vi "Channel Index to Channel Type.vi"(10 "Rx channel range":cluster{"minimum":i32, "maximum":i32}={"minimum"=0, "maximum"=15}, 11 "hardware channel":i32) -> (2 "custom device channel type":T1, 3 "GUID for hardware channel type":string)   [LabVIEW 2020, in "Communication Bus Template Scripting.lvlib"]
uses:
  Communication Bus Template Scripting.lvlib
  <vilib>/NI VeriStand/Custom Device API/Custom Device Channel Type.ctl
  Constants.vi
  <vilib>/NI VeriStand/Custom Device API/Custom Device API.lvlib
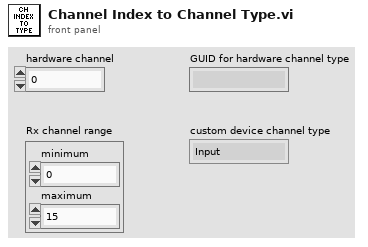
[diagram p1: front panel]
types:
  T1 = typedef "Custom Device API.lvlib/Custom Device Channel Type.ctl" = enum16{"Input", "Output"}
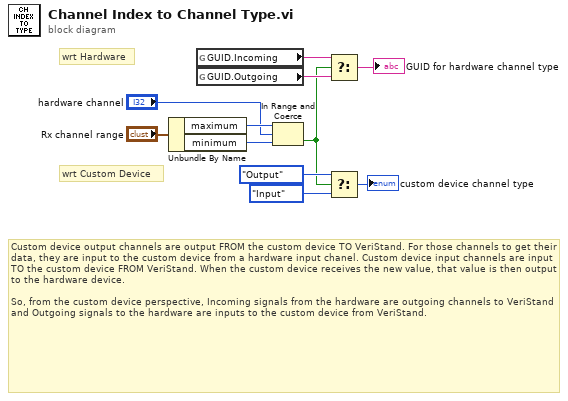
[diagram p0: block diagram]
diagram:
  # "wrt Custom Device"
  # "wrt Hardware"
  # "Custom device output channels are output FROM the custom device TO VeriStand. For those channels to get their data, they are input to the custom device from a hardware input chanel. Custom device input channels are input TO the custom device FROM VeriStand. When the custom device receives the new value, that value is then output to the hardware device.\n \nSo, from the custom device perspective, Incoming signals from the hardware are outgoing channels to VeriStand and Outgoing signals to the hardware are inputs to the custom device from VeriStand."
  n1 = Unbundle By Name("Rx channel range") -> ("maximum"=w7:i32, "minimum"=w6:i32)
  n2 = global read "Constants.vi" "GUID.Incoming"() -> (w4:string)
  n3 = global read "Constants.vi" "GUID.Outgoing"() -> (w3:string)
  n4 = In Range and Coerce(upper limit=w7, x="hardware channel", lower limit=w6) -> (In Range?=w2:bool)  [unwired: 1 out]
  n5 = Select(t=w4, s=w2, f=w3) -> (s? t:f=→"GUID for hardware channel type":string)
  n6 = Select(t=Custom_Device_Channel_Type."Output" ("Type"), s=w2, f=Custom_Device_Channel_Type."Input" ("Type")) -> (s? t:f=→"custom device channel type":T1)
